vi "Plugin Wrapper Subpanel.vi"() -> ()   [LabVIEW 2021, in "CIF Manager UI.lvlib"]
uses:
  CIF Manager UI.lvlib
  CIFUI/Typedef/Run Listen Button.ctl
  CIFUI/Typedef/Class Data for SubPanel.ctl
  <vilib>/gRPC/LabVIEW gRPC Library/Shared/grpcId.ctl
  CIFUI/Typedef/Core UI References.ctl
  CIFUI/Typedef/Channel Connection.ctl
  CIFUI/Typedef/New Plugin.ctl
  CIFUI/Typedef/CIF_Manager_UI_Tab.ctl
  CIFUI/Typedef/SubPanel Events.ctl
  CIFUI/Typedef/New Connection Event Data.ctl
  CIFUI/Typedef/New Connection Plugin Event Data.ctl
  CIFUI/CIF_UI.lvclass
  CIFUI/CIF_UI.lvclass/CIF_UI.ctl
  CIFUI/Utilities/Get Human Readable Error.vi
  <vilib>/CIF Foundation/CIF Utilities/Errors/Append Error Location.vi
  CIFUI/UI Element Update/Empty Tree by Reference.vi
  CIFUI/UI Element Update/Empty Table by Reference.vi
  CIFUI/UI Element Update/Initialize Manager Tab by Reference.vi
  CIFUI/Parent to Subpanel/Close Plugin SubPanel.vi
  CIFUI/SubVIs/Check UI Update Timer.vi
  <vilib>/CIF Foundation/CIF Utilities/Errors/Human Readable Error Message.vi
  CIFCore/Grpc/CIFCoreWrapper/CIFCoreWrapper.lvlib
  <vilib>/gRPC/LabVIEW gRPC Library/grpc-lvsupport-release.lvlib
panel:
  in  "Plugin Selection":u16(ring)
  in  "Run Listen":T1
  in  "Unload":bool
  in  "Refresh Button":bool
  in  "Plugin Status":string[][](table)
  in  "Class Data for SubPanel":T2
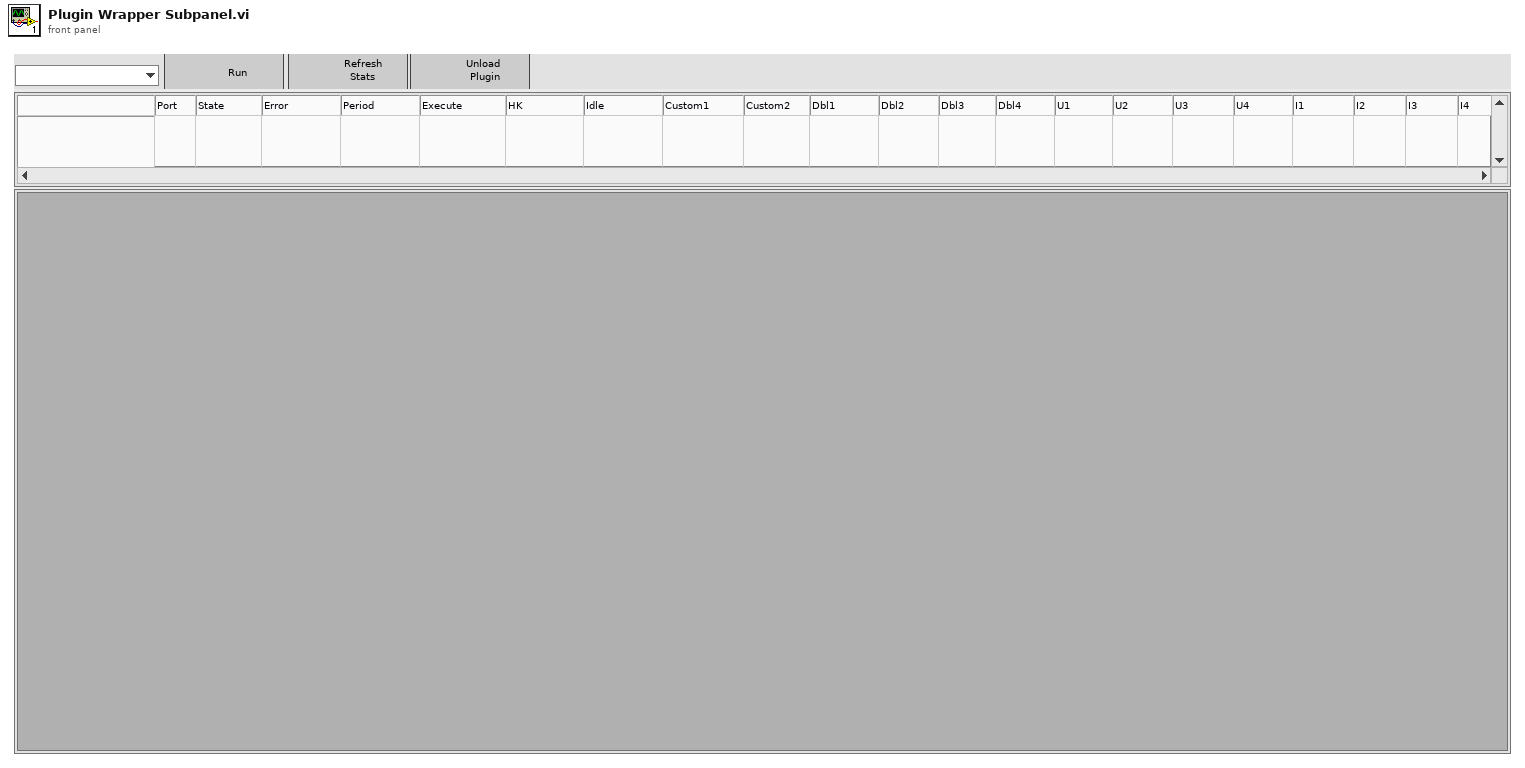
[diagram p1: front panel]
types:
  T1 = typedef "CIF_UI.lvclass/Run Listen Button.ctl" = bool
  T2 = typedef "CIF_UI.lvclass/Class Data for SubPanel.ctl" = cluster{"IP Address":string, "Manager gRPC ID":T3, "Server Certificate File (.crt)":path, "Connected":bool, "Manager Connection":bool, "Core UI References":T4, "Subpanel Events":T5}
  T3 = typedef "grpc-lvsupport-release.lvlib/grpcId.ctl" = u64
  T4 = typedef "CIF_UI.lvclass/Core UI References.ctl" = cluster{"Discovered Plugins":refnum<vi>, "Discovered Plugins Valid":bool, "Loaded Plugins":refnum<vi>, "Loaded Plugins Valid":bool, "Publisher Channels":refnum<vi>, "Publisher Channels Valid":bool, "Subscriber Channels":refnum<vi>, "Subscriber Channels Valid":bool, "Plugin Status":refnum<vi>, "Plugin Status Valid":bool, "Channel Connection":refnum<vi>, "Channel Connection Valid":bool, "New Plugin Load":refnum<vi>, "New Plugin Load Valid":bool, "Errors":refnum<vi>, "Errors Valid":bool, "Plugin to Abort":refnum<vi>, "Plugin to Abort Valid":bool, "Connection":refnum<vi>, "Connection Valid":bool, "Exit":refnum<vi>, "Exit Valid":bool, "Run Listen":refnum<vi>, "Run Listen Valid":bool, "CIF Manager Tab":refnum<vi>, "Manger Tab Valid":bool, "Clear Local Error":refnum<vi>, "Clear Local Error Valid":bool, "Local Error":refnum<vi>, "Local Error Valid":bool, "System Errors":refnum<vi>, "System Errors Valid":bool, "Plugin Selection":refnum<vi>, "Plugin Selection Valid":bool}
  T5 = typedef "CIF_UI.lvclass/SubPanel Events.ctl" = cluster{"Clear Local Error":refnum<user-event>, "Shutdown":refnum<user-event>, "gRPC Connection":refnum<user-event>, "Plugin Connection":refnum<user-event>}
  T6 = typedef "CIF_UI.lvclass/Plugin Connections.ctl" = cluster{"gRPC ID":T3, "Plugin Info":T7}
  T7 = typedef "CIF_UI.lvclass/PluginInfo.ctl" = cluster{"Name":string, "Type":string, "grpc_port":i32, "Version":T8, "Node Status":T9}
  T8 = typedef "CIF_UI.lvclass/Version.ctl" = cluster{"Major":i32, "Minor":i32, "Fix":i32}
  T9 = typedef "CIFCoreCommon.lvlib/gRPC Reported Plugin Status.ctl" = cluster{"State":T10, "Timing Statistics (us)":T11, "FIFO Statistics (us)":T13, "error":T14, "Monitor Doubles":T15, "Monitor U64":T16, "Monitor I64":T17}
  T10 = typedef "CIFCoreCommon.lvlib/Plugin State.ctl" = enum32{"Null", "Creating", "Listening", "Running", "CleaningUp", "Destroying"}
  T11 = typedef "CIFCoreCommon.lvlib/Timing Statistics.ctl" = cluster{"Period":T12, "Wake Error":T12, "Execute":T12, "Housekeep":T12, "Idle":T12, "Cleanup":T12, "Custom 1 (custom units)":T12, "Custom 2 (custom units)":T12}
  T12 = typedef "CIFCoreCommon.lvlib/Timing Stats Base.ctl" = cluster{"Max":i64, "Avg":dbl, "Min":i64}
  T13 = typedef "CIFCoreCommon.lvlib/FIFO Statistics.ctl" = cluster{"From T0":T12, "From Previous Plugin":T12, "Output Error":T12}
  T14 = typedef "CIFCoreCommon.lvlib/Simple Error.ctl" = cluster{"status":bool, "code":i32}
  T15 = typedef "CIFCoreCommon.lvlib/Monitor Doubles.ctl" = cluster{"1":dbl, "2":dbl, "3":dbl, "4":dbl}
  T16 = typedef "CIFCoreCommon.lvlib/Monitor U64.ctl" = cluster{"1":u64, "2":u64, "3":u64, "4":u64}
  T17 = typedef "CIFCoreCommon.lvlib/Monitor I64.ctl" = cluster{"1":i64, "2":i64, "3":i64, "4":i64}
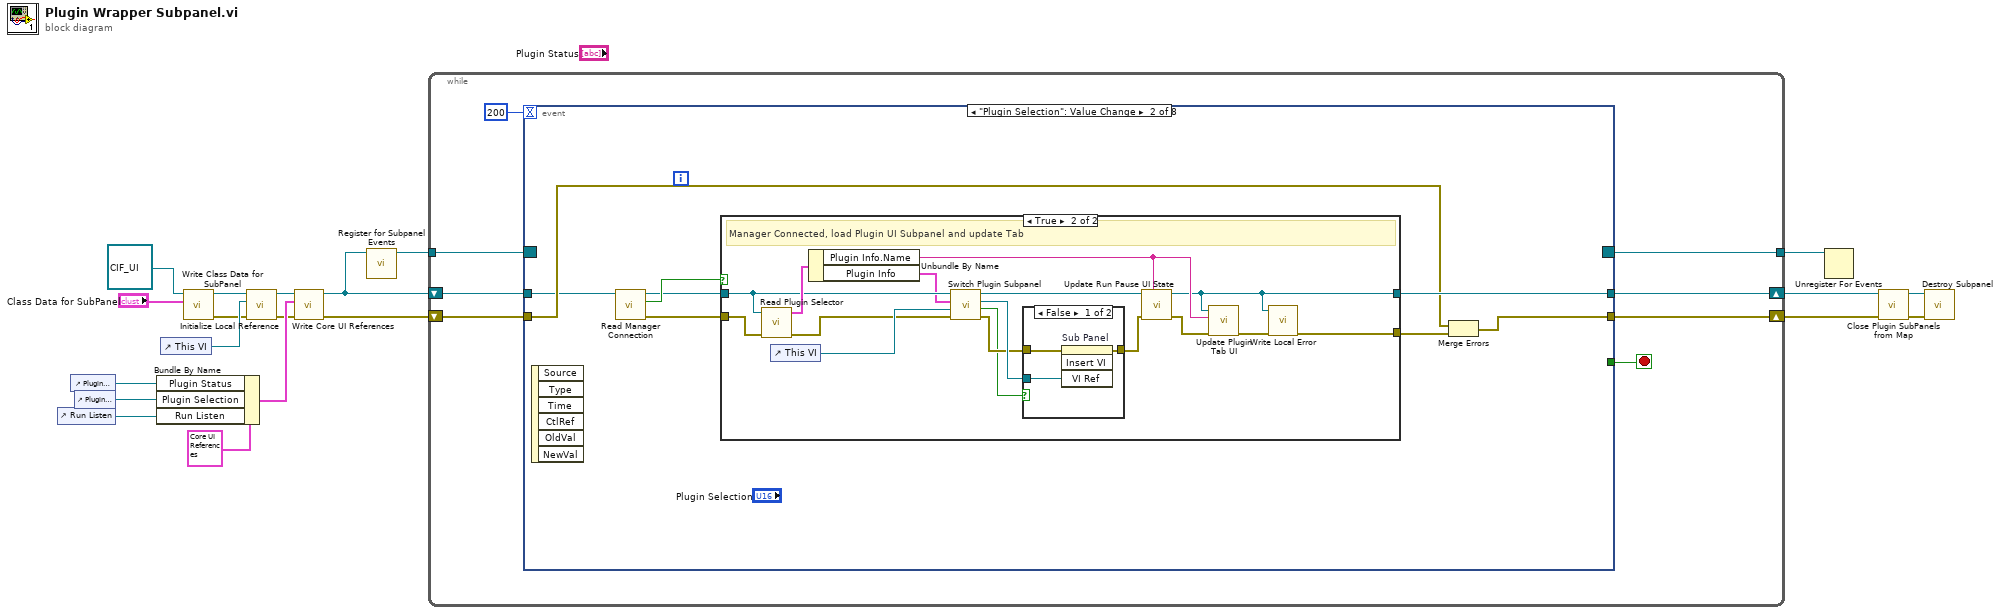
[diagram p0: block diagram]
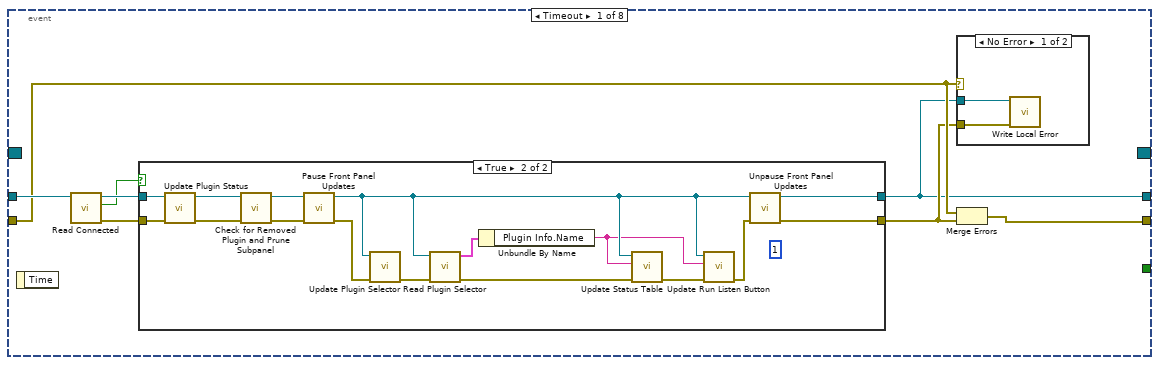
[diagram p2: hidden frame]
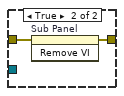
[diagram p6: hidden frame]
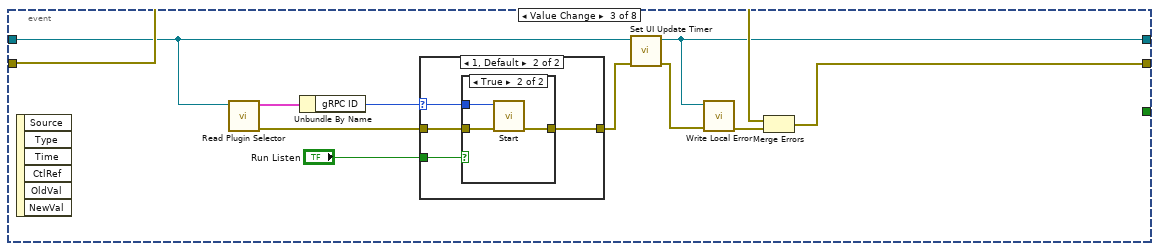
[diagram p7: hidden frame]
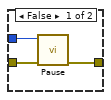
[diagram p9: hidden frame]
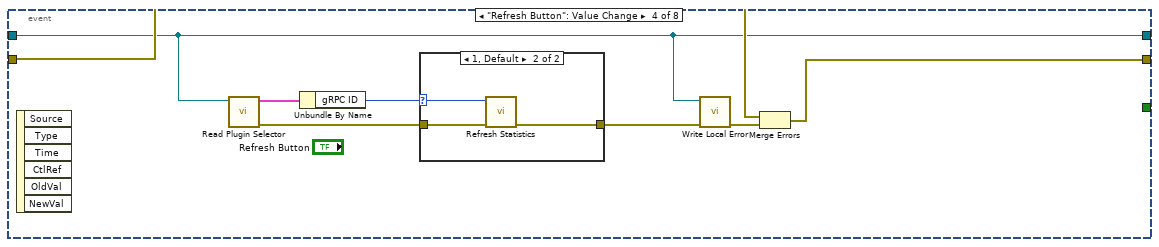
[diagram p10: hidden frame]
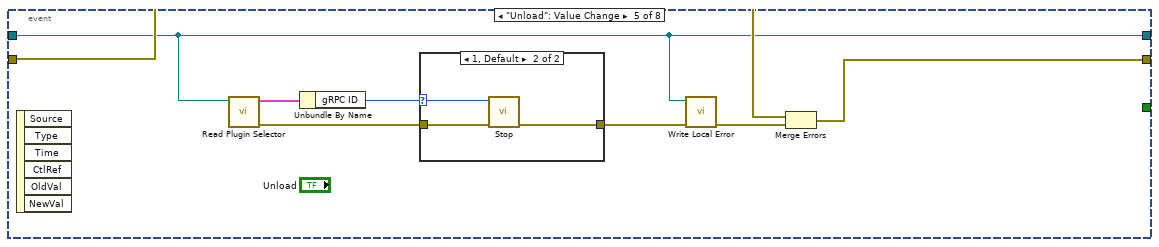
[diagram p12: hidden frame]
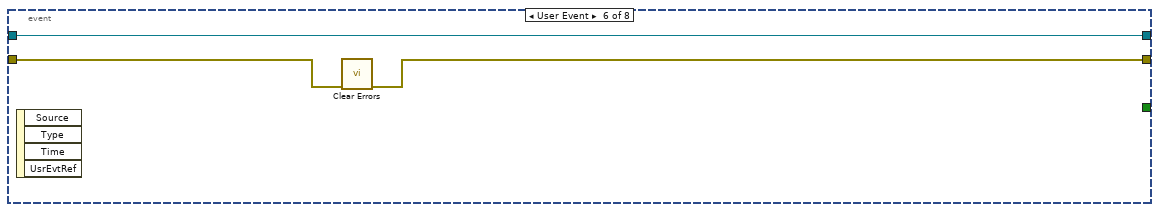
[diagram p14: hidden frame]
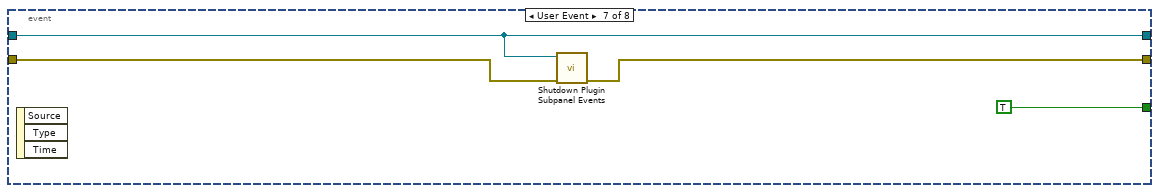
[diagram p15: hidden frame]
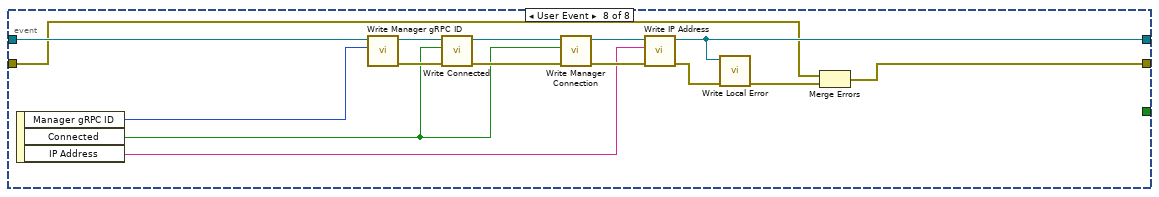
[diagram p16: hidden frame]
diagram:
  n1 = control-ref of="Run Listen"() -> (w10:refnum<vi>)
  n2 = control-ref of="Plugin Status"() -> (w17:refnum<vi>)
  n3 = control-ref of="Plugin Selection"() -> (w11:refnum<vi>)
  n4 = Bundle By Name(cluster=T4 {"Discovered Plugins"=refnum, "Discovered Plugins Valid"=FALSE, "Loaded Plugins"=refnum, "Loaded Plugins Valid"=FALSE, "Publisher Channels"=refnum, "Publisher Channels Valid"=FALSE, "Subscriber Channels"=refnum, "Subscriber Channels Valid"=FALSE, "Plugin Status"=refnum, "Plugin Status Valid"=FALSE, "Channel Connection"=refnum, "Channel Connection Valid"=FALSE, "New Plugin Load"=refnum, "New Plugin Load Valid"=FALSE, "Errors"=refnum, "Errors Valid"=FALSE, "Plugin to Abort"=refnum, "Plugin to Abort Valid"=FALSE, "Connection"=refnum, "Connection Valid"=FALSE, "Exit"=refnum, "Exit Valid"=FALSE, "Run Listen"=refnum, "Run Listen Valid"=FALSE, "CIF Manager Tab"=refnum, "Manger Tab Valid"=FALSE, "Clear Local Error"=refnum, "Clear Local Error Valid"=FALSE, "Local Error"=refnum, "Local Error Valid"=FALSE, "System Errors"=refnum, "System Errors Valid"=FALSE, "Plugin Selection"=refnum, "Plugin Selection Valid"=FALSE} ("UI References"), "Plugin Status"=w17, "Plugin Selection"=w11, "Run Listen"=w10) -> (w18:T4)
  n5 = control-ref of="This VI"() -> (w14:refnum<vi>)
  n6 = call "Write Class Data for SubPanel.vi"("Class Data for SubPanel"="Class Data for SubPanel", "CIF_UI in"=refnum<class "CIF_UI.lvclass"> refnum) -> ("error out"=w3:errorcluster, "CIF_UI out"=w4:refnum<class "CIF_UI.lvclass">)  [unwired: 8 in]
  n7 = call "Initialize Local Reference.vi"("error in (no error)"=w3, "This VI"=w14, "CIF_UI in"=w4) -> ("error out"=w12:errorcluster, "CIF_UI out"=w13:refnum<class "CIF_UI.lvclass">)  [unwired: 7 in]
  n8 = call "Write Core UI References.vi"("error in (no error)"=w12, "UI References"=w18, "CIF_UI in"=w13) -> ("error out"=w19:errorcluster, "CIF_UI out"=w16:refnum<class "CIF_UI.lvclass">)  [unwired: 7 in]
  n9 = call "Register for Subpanel Events.vi"("CIF_UI in"=w16) -> ("Event Registration Refnum"=w15:refnum<event-registration>)  [unwired: 9 in, 1 out]
  n10 = while {
    shift-right: [w24] -> w9
    shift-left: w16 -> [w26]
    shift-right: [w21] -> w1
    shift-left: w19 -> [w25]
    tunnel: w15 -> [w23]
    tunnel: [w22] -> w2
    stop <- w27 stop-if-true
    n11 = event shown="[1] \"Plugin Selection\": Value Change" {
      selector: w23 -> [_ _ _ _ _ _ _ _]
      dyn-events: [_ _ _ _ _ _ _ _] -> w22
      timeout: 200 -> [_ _ _ _ _ _ _ _]
      tunnel: [_ _ _ _ _ _ TRUE _] -> w27
      tunnel: w26 -> [w33 w58 w91 w110 w122 w134 w139 w149]
      tunnel: w25 -> [w32 w60 w93 w111 w124 w136 w138 w143]
      tunnel: [w30 w59 w92 w112 w123 w135 w137 w142] -> w21
      tunnel: [w29 w61 w90 w110 w122 w134 w139 w144] -> w24
      event Timeout {
        n12 = event-data() -> ()  [unwired: 1 in, 1 out]
        n13 = call "Read Connected.vi"("CIF_UI in"=w33) -> ("error out"=w35:errorcluster, "Connected"=w34:bool, "CIF_UI out"=w36:refnum<class "CIF_UI.lvclass">)  [unwired: 8 in]
        n14 = case shown="True" w34 {
          tunnel: w35 -> [w39 w56]
          tunnel: [w39 w41] -> w31
          tunnel: w36 -> [w40 w55]
          tunnel: [w40 w42] -> w29
          frame False {
          }
          frame True {
            (unwired) 1 ("code")
            n15 = call "Update Plugin Status.vi"("error in (no error)"=w56, "CIF_UI in"=w55) -> ("error out"=w52:errorcluster, "CIF_UI out"=w53:refnum<class "CIF_UI.lvclass">)  [unwired: 8 in]
            n16 = call "Check for Removed Plugin and Prune Subpanel.vi"("error in (no error)"=w52, "CIF_UI in"=w53) -> ("error out"=w50:errorcluster, "CIF_UI out"=w51:refnum<class "CIF_UI.lvclass">)  [unwired: 8 in]
            n17 = call "Pause Front Panel Updates.vi"("error in (no error)"=w50, "CIF_UI in"=w51) -> ("error out"=w48:errorcluster, "CIF_UI out"=w44:refnum<class "CIF_UI.lvclass">)  [unwired: 8 in]
            n18 = call "Update Plugin Selector.vi"("error in (no error)"=w48, "CIF_UI in"=w44) -> ("error out"=w49:errorcluster)  [unwired: 9 in]
            n19 = call "Read Plugin Selector.vi"("error in (no error)"=w49, "CIF_UI in"=w44) -> ("error out"=w47:errorcluster, "Plugin Info"=w54:T6)  [unwired: 8 in]
            n20 = Unbundle By Name(w54) -> ("Plugin Info.Name"=w43:string)
            n21 = call "Update Status Table.vi"("error in (no error)"=w47, "Plugin Filter"=w43, "CIFManager_UI in"=w44) -> ("error out"=w46:errorcluster)  [unwired: 8 in]
            n22 = call "Update Run Listen Button.vi"("error in (no error)"=w46, "Plugin Filter"=w43, "CIFManager_UI in"=w44) -> ("error out"=w45:errorcluster)  [unwired: 8 in]
            n23 = call "Unpause Front Panel Updates.vi"("error in (no error)"=w45, "CIF_UI in"=w44) -> ("error out"=w41:errorcluster, "CIF_UI out"=w42:refnum<class "CIF_UI.lvclass">)  [unwired: 8 in]
          }
        }
        n24 = case shown="No Error" w32 {
          tunnel: w29 -> [w38 _]
          tunnel: w31 -> [w37 _]
          frame No Error {
            n25 = call "Write Local Error.vi"("error in (no error)"=w37, "CIF_UI in"=w38) -> ()  [unwired: 9 in, 1 out]
          }
          frame Error {
          }
        }
        n26 = Merge Errors(w32, w31) -> (w30:errorcluster)
      }
      event "Plugin Selection": Value Change {
        n27 = event-data() -> ()  [unwired: 1 in, 6 out]
        n28 = call "Read Manager Connection.vi"("CIF_UI in"=w58) -> ("error out"=w62:errorcluster, "Manager Connection"=w64:bool, "CIF_UI out"=w63:refnum<class "CIF_UI.lvclass">)  [unwired: 8 in]
        n29 = case shown="True" w64 {
          tunnel: w62 -> [w65 w82]
          tunnel: w63 -> [w66 w79]
          tunnel: [w66 w71] -> w61
          tunnel: [w65 w70] -> w57
          frame False {
            # "Manager not connected.  Input is not valid. Skip"
          }
          frame True {
            # "Manager Connected, load Plugin UI Subpanel and update Tab"
            n30 = call "Read Plugin Selector.vi"("error in (no error)"=w82, "CIF_UI in"=w79) -> ("error out"=w68:errorcluster, "Plugin Info"=w80:T6)  [unwired: 8 in]
            n31 = control-ref of="This VI"() -> (w73:refnum<vi>)
            n32 = Unbundle By Name(w80) -> ("Plugin Info.Name"=w76:string, "Plugin Info"=w74:T7)
            n33 = call "Switch Plugin Subpanel.vi"("error in (no error)"=w68, "Calling VI"=w73, "Plugin Info"=w74, "CIF_UI in"=w79) -> ("error out"=w69:errorcluster, "Remove Subpanel"=w67:bool, "VI Reference"=w81:refnum<vi>, "CIF_UI out"=w75:refnum<class "CIF_UI.lvclass">)  [unwired: 4 in]
            n34 = case shown="False" w67 {
              tunnel: w81 -> [w85 _]
              tunnel: [w84 w86] -> w78
              tunnel: w69 -> [w83 w87]
              frame False {
                n35 = invoke on="Sub Panel" class="SubPnl" method="Insert VI"(error in=w83, "VI Ref"=w85) -> (error out=w84:errorcluster)  [unwired: 2 in, 3 out]
              }
              frame True {
                n36 = invoke on="Sub Panel" class="SubPnl" method="Remove VI"(error in=w87) -> (error out=w86:errorcluster)  [unwired: 2 in, 2 out]
              }
            }
            n37 = call "Update Run Pause UI State.vi"("Plugin Name"=w76, "error in (no error)"=w78, "CIF_UI in"=w75) -> ("error out"=w77:errorcluster, "CIF_UI out"=w71:refnum<class "CIF_UI.lvclass">)  [unwired: 7 in]
            n38 = call "Update Plugin Tab UI.vi"("error in (no error)"=w77, "Plugin Name"=w76, "CIF_UI in"=w71) -> ("error out"=w72:errorcluster)  [unwired: 8 in]
            n39 = call "Write Local Error.vi"("error in (no error)"=w72, "CIF_UI in"=w71) -> ("error out"=w70:errorcluster)  [unwired: 9 in]
          }
        }
        n40 = Merge Errors(w60, w57) -> (w59:errorcluster)
      }
      event Value Change {
        n41 = event-data() -> ()  [unwired: 1 in, 6 out]
        n42 = call "Read Plugin Selector.vi"("CIF_UI in"=w91) -> ("error out"=w96:errorcluster, "Plugin Info"=w98:T6)  [unwired: 9 in]
        n43 = Unbundle By Name(w98) -> ("gRPC ID"=w97:T3)
        n44 = case shown="1, Default" w97 {
          selector: w97 -> [_ w103]
          tunnel: w96 -> [w99 w102]
          tunnel: "Run Listen" -> [_ w101]
          tunnel: [w99 w100] -> w89
          frame 0 {
          }
          frame 1, Default {
            n45 = case shown="True" w101 {
              tunnel: w103 -> [w106 w109]
              tunnel: w102 -> [w105 w108]
              tunnel: [w104 w107] -> w100
              frame False {
                n46 = call "Pause.vi"("error in"=w105, "gRPC ID"=w106) -> ("error out"=w104:errorcluster)  [unwired: 8 in, 1 out]
              }
              frame True {
                n47 = call "Start.vi"("error in"=w108, "gRPC ID"=w109) -> ("error out"=w107:errorcluster)  [unwired: 8 in, 1 out]
              }
            }
          }
        }
        n48 = call "Set UI Update Timer.vi"("error in (no error)"=w89, "CIF_UI in"=w91) -> ("error out"=w88:errorcluster, "CIF_UI out"=w90:refnum<class "CIF_UI.lvclass">)  [unwired: 8 in]
        n49 = call "Write Local Error.vi"("error in (no error)"=w88, "CIF_UI in"=w90) -> ("error out"=w94:errorcluster)  [unwired: 9 in]
        n50 = Merge Errors(w93, w94) -> (w92:errorcluster)
      }
      event "Refresh Button": Value Change {
        n51 = event-data() -> ()  [unwired: 1 in, 6 out]
        n52 = call "Read Plugin Selector.vi"("CIF_UI in"=w110) -> ("error out"=w115:errorcluster, "Plugin Info"=w117:T6)  [unwired: 9 in]
        n53 = Unbundle By Name(w117) -> ("gRPC ID"=w116:T3)
        n54 = case shown="1, Default" w116 {
          selector: w116 -> [_ w121]
          tunnel: w115 -> [w118 w120]
          tunnel: [w118 w119] -> w114
          frame 0 {
          }
          frame 1, Default {
            n55 = call "Refresh Statistics.vi"("error in"=w120, "gRPC ID"=w121) -> ("error out"=w119:errorcluster)  [unwired: 8 in, 1 out]
          }
        }
        n56 = call "Write Local Error.vi"("error in (no error)"=w114, "CIF_UI in"=w110) -> ("error out"=w113:errorcluster)  [unwired: 9 in]
        n57 = Merge Errors(w111, w113) -> (w112:errorcluster)
      }
      event "Unload": Value Change {
        n58 = event-data() -> ()  [unwired: 1 in, 6 out]
        n59 = call "Read Plugin Selector.vi"("CIF_UI in"=w122) -> ("error out"=w127:errorcluster, "Plugin Info"=w129:T6)  [unwired: 9 in]
        n60 = Unbundle By Name(w129) -> ("gRPC ID"=w128:T3)
        n61 = case shown="1, Default" w128 {
          selector: w128 -> [_ w131]
          tunnel: w127 -> [w130 w133]
          tunnel: [w130 w132] -> w126
          frame 0 {
          }
          frame 1, Default {
            n62 = call "Stop.vi"("error in"=w133, "gRPC ID"=w131) -> ("error out"=w132:errorcluster)  [unwired: 8 in, 1 out]
          }
        }
        n63 = call "Write Local Error.vi"("error in (no error)"=w126, "CIF_UI in"=w122) -> ("error out"=w125:errorcluster)  [unwired: 9 in]
        n64 = Merge Errors(w124, w125) -> (w123:errorcluster)
      }
      event User Event {
        n65 = event-data() -> ()  [unwired: 1 in, 4 out]
        n66 = call <vilib>:"Clear Errors.vi"("error in (no error)"=w136) -> ("error out"=w135:errorcluster)  [unwired: 5 in, 1 out]
      }
      event User Event {
        n67 = event-data() -> ()  [unwired: 1 in, 3 out]
        n68 = call "Shutdown Plugin Subpanel Events.vi"("error in (no error)"=w138, "CIF_UI in"=w139) -> ("error out"=w137:errorcluster)  [unwired: 9 in]
      }
      event User Event {
        n69 = event-data() -> ("Manager gRPC ID"=w146:T3, "Connected"=w147:bool, "IP Address"=w148:string)  [unwired: 1 in]
        n70 = call "Write Manager gRPC ID.vi"("gRPCid"=w146, "CIF_UI in"=w149) -> ("error out"=w154:errorcluster, "CIF_UI out"=w155:refnum<class "CIF_UI.lvclass">)  [unwired: 8 in]
        n71 = call "Write Connected.vi"("error in (no error)"=w154, "Connected"=w147, "CIF_UI in"=w155) -> ("error out"=w152:errorcluster, "CIF_UI out"=w153:refnum<class "CIF_UI.lvclass">)  [unwired: 7 in]
        n72 = call "Write Manager Connection.vi"("error in (no error)"=w152, "Manager Connection"=w147, "CIF_UI in"=w153) -> ("error out"=w150:errorcluster, "CIF_UI out"=w151:refnum<class "CIF_UI.lvclass">)  [unwired: 7 in]
        n73 = call "Write IP Address.vi"("error in (no error)"=w150, "IP Address"=w148, "CIF_UI in"=w151) -> ("error out"=w145:errorcluster, "CIF_UI out"=w144:refnum<class "CIF_UI.lvclass">)  [unwired: 7 in]
        n74 = call "Write Local Error.vi"("error in (no error)"=w145, "CIF_UI in"=w144) -> ("error out"=w141:errorcluster)  [unwired: 9 in]
        n75 = Merge Errors(w143, w141) -> (w142:errorcluster)
      }
    }
  }
  n76 = Unregister For Events(event registration refnum=w2) -> ()  [unwired: 1 in, 1 out]
  n77 = call "Close Plugin SubPanels from Map.vi"("error in (no error)"=w1, "CIF_UI in"=w9) -> ("error out"=w8:errorcluster, "CIF_UI out"=w7:refnum<class "CIF_UI.lvclass">)  [unwired: 8 in]
  n78 = call "Destroy Subpanel.vi"("error in (no error)"=w8, "CIF_UI in"=w7) -> ()  [unwired: 8 in, 2 out]
